vi "WPI_AnalogChannelGetVoltage.vi"(8 "error in (no error)":errorcluster, 11 "AIDeviceRef":T1={"DevStatus"={"status"=FALSE, "code"=0, "source"=""}, "Analog Channel"=enum."Invalid"}) -> (0 "error out":errorcluster, 2 "Voltage":dbl, 3 "AIDeviceRef":T1={"DevStatus"={"status"=FALSE, "code"=0, "source"=""}, "Analog Channel"=enum."Invalid"})   [LabVIEW 2017]
doc: "Returns the voltage value directly from the A/D converter on the channel. The converter scales the raw value to the voltage value using the least significant bit weight constant and the offset constant of the hardware. Use the GetAverageVoltage VI to get voltage values from oversampled or averaged signals.\n\nThis software is licensed. Open the labview\\readme\\WPI Robotics Library Open Source License.txt file for more information."
uses:
  <vilib>/Rock Robotics/WPI/AnalogChannel/WPI_AnalogChannelDevRef.ctl
  <vilib>/Rock Robotics/SystemInterfaces/AI/FPGA_AIChannel.ctl
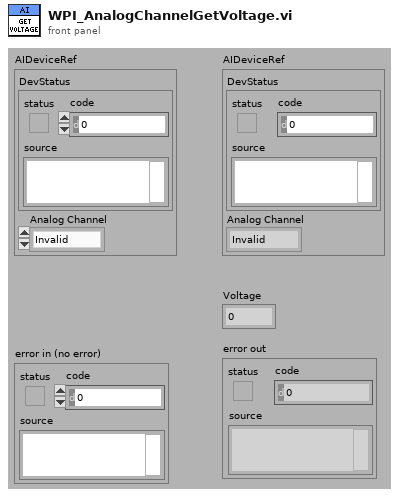
[diagram p1: front panel]
types:
  T1 = typedef "WPI_AnalogChannelDevRef.ctl" = cluster{"DevStatus":errorcluster, "Analog Channel":T2}
  T2 = typedef "FPGA_AIChannel.ctl" = enum8{"AI 0", "AI 1", "AI 2", "AI 3", "AI MXP 0", "AI MXP 1", "AI MXP 2", "AI MXP 3", "Invalid"}
  T3 = typedef "WPI_AnalogModuleDevStatus.ctl" = cluster{"DevStatus":errorcluster}
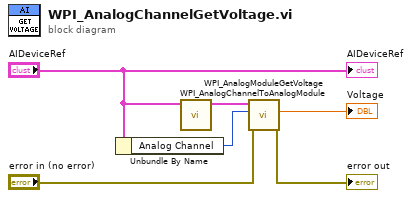
[diagram p0: block diagram]
diagram:
  n1 = Unbundle By Name("AIDeviceRef") -> ("Analog Channel"=w5:T2)
  n2 = call <vilib>:"WPI_AnalogChannelToAnalogModule.vi"("AIDeviceRef"="AIDeviceRef") -> ("AIDeviceRef"=w4:T3)  [unwired: 10 out]
  n3 = call <vilib>:"WPI_AnalogModuleGetVoltage.vi"("error in (no error)"="error in (no error)", "Channel"=w5, "AnalogModuleDevRef"=w4) -> ("error out"=→"error out":errorcluster, "Voltage"=→"Voltage":dbl)  [unwired: 7 out]
  "AIDeviceRef" <- "AIDeviceRef"
